vi "RobotAndM4Title整合.vi"(0 "RobotTielte":string[](array[string])) -> (7 "Title数据整合输出":string[](array[string]))   [LabVIEW 2011]
panel:
  # "Product\nStationID\nMachineSN\nHW\nGUI-Ver\nRobot-Ver\nVision-Ver\nIP\nMachinMAC\nPointX\t\nPointY\t\nAngle\nStartTime\nEndTime\nTime of CCD photographing\nM4 FPYR\t\nM4 Failing Rate\nM4 ReTest\nM4 CumRetestYield\nM4 ThroughtRate\nRobot-OriginPosition\t\nRobot-CCD TopPosition"
  # "SN\nM4 Result\nblack wifiˊ0.0\nM4 Fixture 1\nErrorCode"
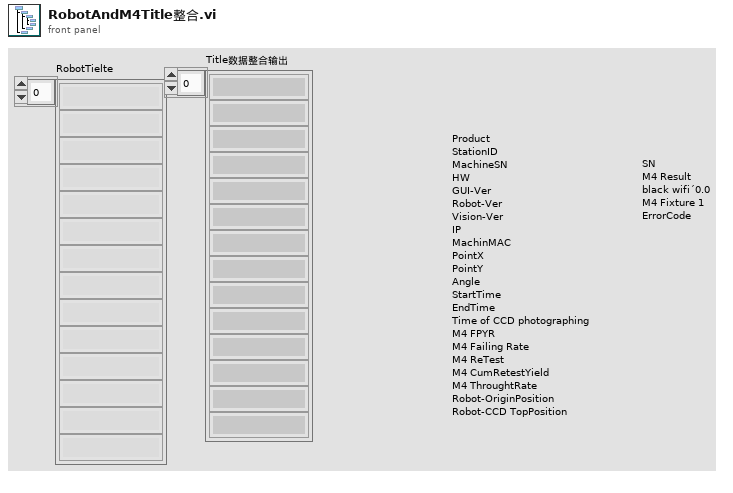
[diagram p1: front panel]
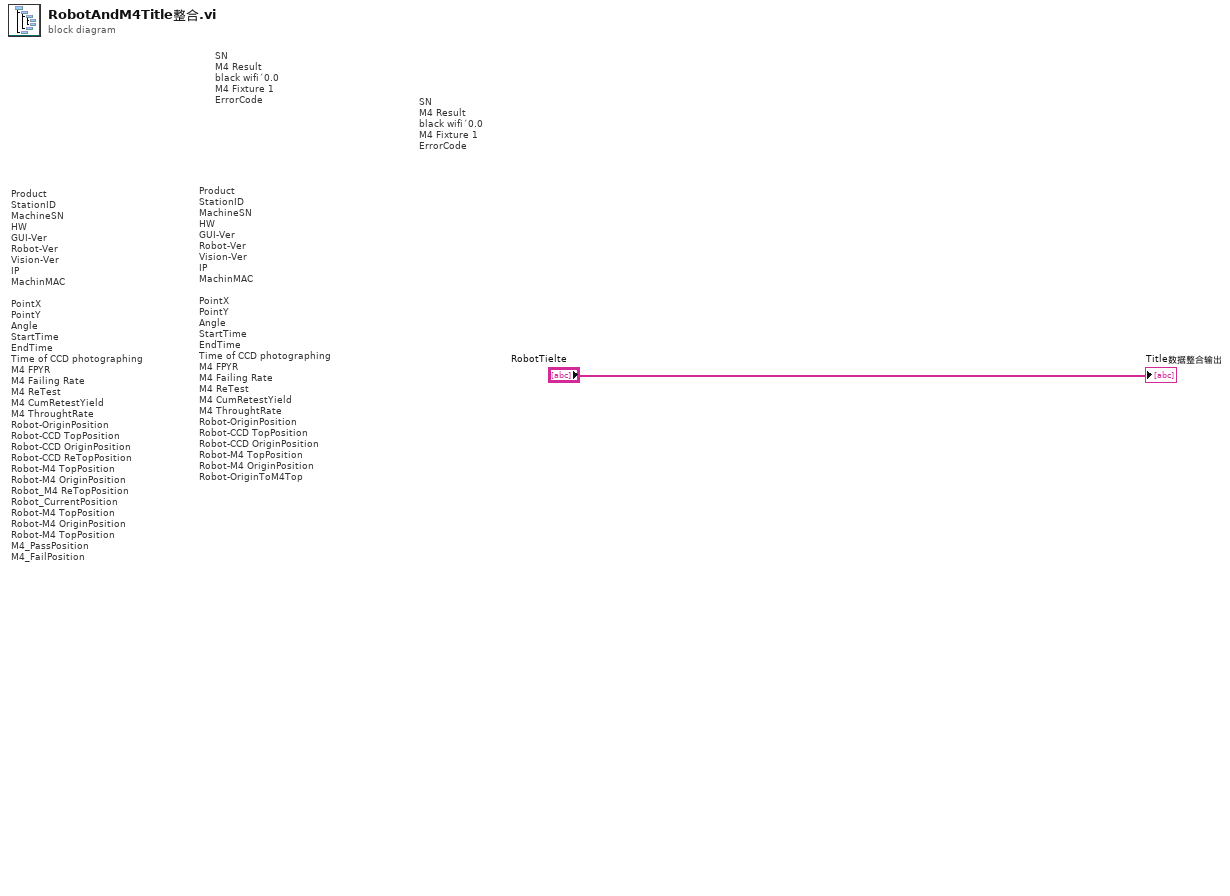
[diagram p0: block diagram]
diagram:
  # "Product\nStationID\nMachineSN\nHW\nGUI-Ver\nRobot-Ver\nVision-Ver\nIP\nMachinMAC\n\nPointX\t\nPointY\t\nAngle\nStartTime\nEndTime\nTime of CCD photographing\nM4 FPYR\t\nM4 Failing Rate\nM4 ReTest\nM4 CumRetestYield\nM4 ThroughtRate\nRobot-OriginPosition\t\nRobot-CCD TopPosition\t\nRobot-CCD OriginPosition\nRobot-CCD ReTopPosition\t\nRobot-M4 TopPosition\t\nRobot-M4 OriginPosition\t\nRobot_M4 ReTopPosition\nRobot_CurrentPosition\nRobot-M4 TopPosition\nRobot-M4 OriginPosition\t\nRobot-M4 TopPosition\nM4_PassPosition\nM4_FailPosition"
  # "SN\nM4 Result\nblack wifiˊ0.0\nM4 Fixture 1\nErrorCode"
  # "SN\nM4 Result\nblack wifiˊ0.0\nM4 Fixture 1\nErrorCode"
  # "Product\nStationID\nMachineSN\nHW\nGUI-Ver\nRobot-Ver\nVision-Ver\nIP\nMachinMAC\n\nPointX\t\nPointY\t\nAngle\nStartTime\nEndTime\nTime of CCD photographing\nM4 FPYR\t\nM4 Failing Rate\nM4 ReTest\nM4 CumRetestYield\nM4 ThroughtRate\nRobot-OriginPosition\t\nRobot-CCD TopPosition\t\nRobot-CCD OriginPosition\t\nRobot-M4 TopPosition\t\nRobot-M4 OriginPosition\t\nRobot-OriginToM4Top"
  "Title数据整合输出" <- "RobotTielte"
